vi "I2C Channels.vi"(8 "Error In":errorcluster, 9 "Channel State":T1, 10 "Channel Number":u8, 11 "I2C Channel":variant) -> (0 "Error Out":errorcluster, 3 "I2C Channel":variant)   [LabVIEW 2014, in "LMH-LINX.lvlib"]
doc: "Functional Global Variable used to store LINX I2C channels."
uses:
  <vilib>/MakerHub/LINX/LMH-LINX.lvlib
  <vilib>/MakerHub/LINX/Private/Type Defs/Channel FGV States.ctl
panel:
  # "I2C Channel FGV"
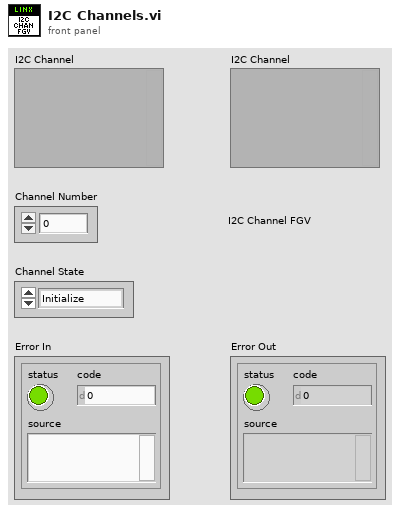
[diagram p1: front panel]
types:
  T1 = typedef "LMH-LINX.lvlib/Channel FGV States.ctl" = enum16{"Initialize", "Get", "Set"}
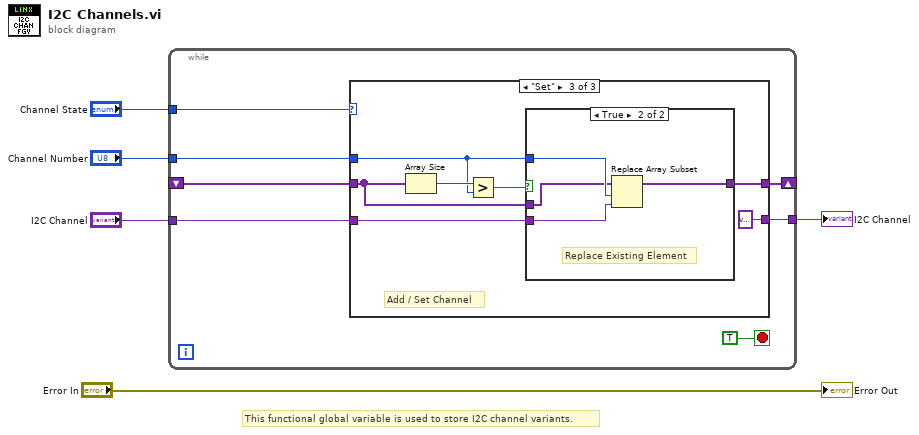
[diagram p0: block diagram]
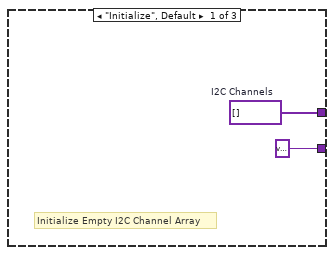
[diagram p2: hidden frame]
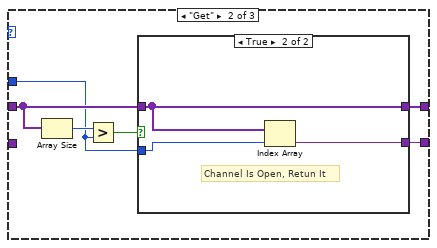
[diagram p3: hidden frame]
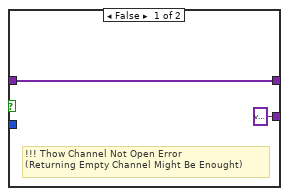
[diagram p4: hidden frame]
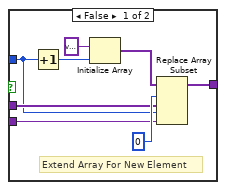
[diagram p5: hidden frame]
diagram:
  # "This functional global variable is used to store I2C channel variants."
  n1 = while {
    shift-right: [w11] -> _
    shift-left: _ -> [w9]
    tunnel: "Channel State" -> [w10]
    tunnel: "Channel Number" -> [w8]
    tunnel: [w7] -> w3
    tunnel: "I2C Channel" -> [w6]
    stop <- TRUE stop-if-true
    n2 = case shown="\"Set\"" w10 {
      tunnel: [w14 w15 w28] -> w11
      tunnel: w9 -> [_ w20 w30]
      tunnel: w8 -> [_ w17 w27]
      tunnel: [variant ("Variant") w16 variant ("I2C Channel")] -> w7
      tunnel: w6 -> [_ _ w29]
      frame "Initialize", Default {
        w14 = variant[] []  # I2C Channels
        # "Initialize Empty I2C Channel Array"
      }
      frame "Get" {
        n3 = Array Size(array=w20) -> (size(s)=w19:i32)
        n4 = Greater?(x=w19, y=w17) -> (0:w18:bool)
        n5 = case shown="True" w18 {
          tunnel: w20 -> [w21 w23]
          tunnel: w17 -> [_ w25]
          tunnel: [variant ("Variant") w24] -> w16
          tunnel: [w21 w23] -> w15
          frame False {
            # "!!! Thow Channel Not Open Error\n(Returning Empty Channel Might Be Enought)"
          }
          frame True {
            # "Channel Is Open, Retun It"
            n6 = Index Array(array=w23, index=w25) -> (element=w24:variant)
          }
        }
      }
      frame "Set" {
        # "Add / Set Channel"
        n7 = Array Size(array=w30) -> (size(s)=w31:i32)
        n8 = Greater?(x=w31, y=w27) -> (0:w32:bool)
        n9 = case shown="True" w32 {
          tunnel: [w36 w44] -> w28
          tunnel: w27 -> [w34 w43]
          tunnel: w30 -> [w38 w42]
          tunnel: w29 -> [w37 w41]
          frame False {
            # "Extend Array For New Element"
            n10 = Increment(x=w34) -> (x+1=w35:u8)
            n11 = Initialize Array(variant ("I2C Channel"), w35) -> (w40:variant[])
            n12 = Replace Array Subset(array=w40, new element #1=w38, index #1=0 ("index"), new element #2=w37, index #2=w34) -> (w36:variant[])
          }
          frame True {
            # "Replace Existing Element"
            n13 = Replace Array Subset(array=w42, new element=w41, index=w43) -> (w44:variant[])
          }
        }
      }
    }
  }
  "I2C Channel" <- w3
  "Error Out" <- "Error In"
